vi "Create chained opcode.vi"(9 "new cmd opcode":string, 10 "Number of commands":dbl, 11 "Current cmd opcode":string) -> (3 "new chained opcode":string)   [LabVIEW 2020]
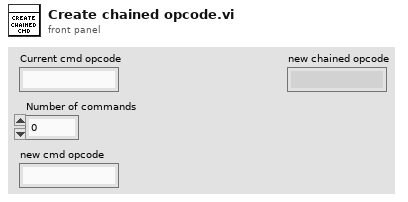
[diagram p1: front panel]
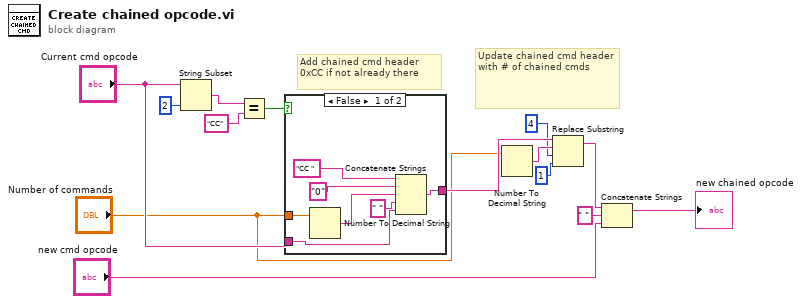
[diagram p0: block diagram]
diagram:
  # "Update chained cmd header with # of chained cmds"
  # "Add chained cmd header 0xCC if not already there"
  n1 = String Subset(string="Current cmd opcode", length (rest)=2 ("length (rest)")) -> (substring=w12:string)  [unwired: 1 in]
  n2 = Equal?(x=w12, y="CC") -> (x = y?=w10:bool)
  n3 = case shown="False" w10 {
    tunnel: [w21 w22] -> w6
    tunnel: "Number of commands" -> [w18 _]
    tunnel: "Current cmd opcode" -> [w15 w22]
    frame False {
      n4 = Number To Decimal String(number=w18) -> (decimal integer string=w17:string)  [unwired: 1 in]
      n5 = Concatenate Strings("CC " ("string"), "0" ("string"), w17, " " ("string"), w15) -> (w21:string)
    }
    frame True {
    }
  }
  n6 = Number To Decimal String(number="Number of commands") -> (decimal integer string=w4:string)  [unwired: 1 in]
  n7 = Replace Substring(2:1 ("length (len. of substring)"), 3:4 ("offset (0)"), 4:w4, 5:w6) -> (1:w1:string)  [unwired: 1 out]
  n8 = Concatenate Strings(w1, " " ("string"), "new cmd opcode") -> (→"new chained opcode":string)
